vi "CalcControl.vi"(4 "Multiplier":dbl=1.0, 5 "Change Brake":dbl=0.02, 6 "Change Throttle":dbl=0.02, 7 "Current Speed":dbl format="%#_13g", 8 "Set Speed":dbl=1.0 format="%#_13g", 9 "Deadzone":dbl=0.01 format="%#_13g", 10 "Current Brake":dbl=0.5499999999999999 format="%#_13g", 11 "Current Throttle":dbl=0.45 format="%#_13g") -> (1 "Change?":bool=TRUE, 2 "New Brake":dbl=0.49999999999999994 format="%#_13g", 3 "New Throttle":dbl=0.5 format="%#_13g")   [LabVIEW 2014]
panel:
  out "NaN/Path/Refnum?":bool
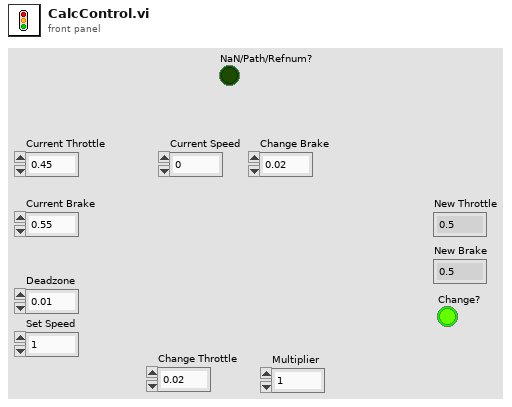
[diagram p1: front panel]
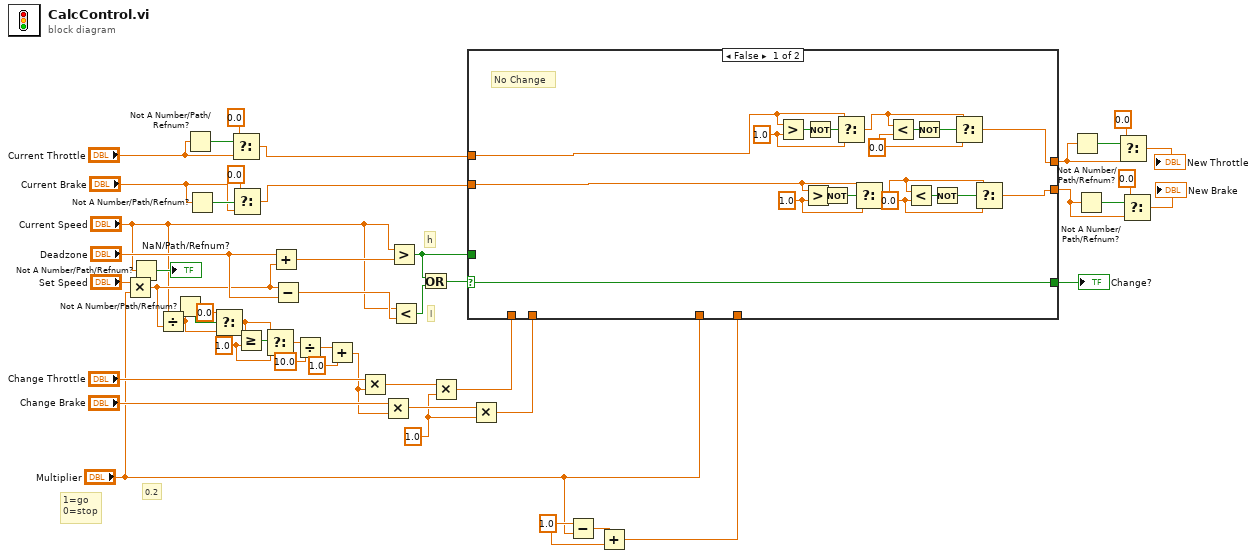
[diagram p0: block diagram]
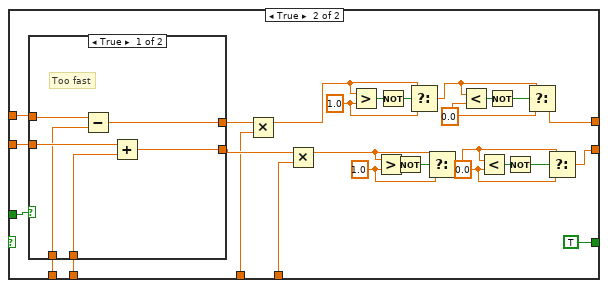
[diagram p2: hidden frame]
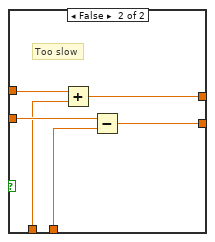
[diagram p3: hidden frame]
diagram:
  w26 = 1.0 ("y")
  w28 = 1.0 ("x")
  w40 = 1.0 ("y")
  # "0.2"
  # "1=go\n0=stop"
  # "l"
  # "h"
  n1 = Multiply(x="Set Speed", y="Multiplier") -> (x*y=w25:dbl)
  n2 = Not A Number/Path/Refnum?(number/path/refnum="Current Speed") -> (NaN/Path/Refnum?=→"NaN/Path/Refnum?":bool)
  n3 = Divide(x="Current Speed", y=w25) -> (x/y=w21:dbl)
  n4 = Not A Number/Path/Refnum?(number/path/refnum=w21) -> (NaN/Path/Refnum?=w23:bool)
  n5 = Not A Number/Path/Refnum?(number/path/refnum="Current Throttle") -> (NaN/Path/Refnum?=w19:bool)
  n6 = Not A Number/Path/Refnum?(number/path/refnum="Current Brake") -> (NaN/Path/Refnum?=w18:bool)
  n7 = Select(t=0.0, s=w23, f=w21) -> (s? t:f=w22:dbl)
  n8 = Select(t=0.0, s=w19, f="Current Throttle") -> (s? t:f=w14:dbl)
  n9 = Select(t=0.0, s=w18, f="Current Brake") -> (s? t:f=w16:dbl)
  n10 = Greater Or Equal?(x=w22, y=w40) -> (x >= y?=w39:bool)
  n11 = Select(t=w22, s=w39, f=w40) -> (s? t:f=w37:dbl)
  n12 = Add(x="Deadzone", y=w25) -> (x+y=w48:dbl)
  n13 = Subtract(x=w25, y="Deadzone") -> (x-y=w47:dbl)
  n14 = Divide(x=w37, y=10.0) -> (x/y=w38:dbl)
  n15 = Add(x=w38, y=1.0) -> (x+y=w34:dbl)
  n16 = Multiply(x="Change Throttle", y=w34) -> (x*y=w31:dbl)
  n17 = Multiply(x="Change Brake", y=w34) -> (x*y=w33:dbl)
  n18 = Greater?(x="Current Speed", y=w48) -> (0:w44:bool)
  n19 = Less?(x="Current Speed", y=w47) -> (x < y?=w46:bool)
  n20 = Or(x=w44, y=w46) -> (x .or. y?=w45:bool)
  n21 = Multiply(x=w31, y=w26) -> (x*y=w30:dbl)
  n22 = Multiply(x=w33, y=w26) -> (x*y=w32:dbl)
  n23 = Subtract(x=w28, y="Multiplier") -> (x-y=w29:dbl)
  n24 = Add(x=w29, y=w28) -> (x+y=w27:dbl)
  n25 = case shown="False" w45 {
    selector: w45 -> [w68 _]
    tunnel: w44 -> [_ w96]
    tunnel: w14 -> [w52 w95]
    tunnel: w16 -> [w53 w94]
    tunnel: w30 -> [_ w93]
    tunnel: [w51 w75] -> w3
    tunnel: [w50 w74] -> w4
    tunnel: [w68 TRUE] -> w43
    tunnel: w32 -> [_ w73]
    tunnel: w27 -> [_ w70]
    tunnel: "Multiplier" -> [_ w69]
    frame False {
      w62 = 0.0 ("y")
      w61 = 1.0 ("y")
      w65 = 0.0 ("y")
      w66 = 1.0 ("y")
      # "No Change"
      n26 = Greater?(x=w52, y=w66) -> (0:w67:bool)
      n27 = Greater?(x=w53, y=w61) -> (0:w60:bool)
      n28 = Not(x=w67) -> (.not. x?=w54:bool)
      n29 = Not(x=w60) -> (.not. x?=w56:bool)
      n30 = Select(t=w52, s=w54, f=w66) -> (s? t:f=w58:dbl)
      n31 = Select(t=w53, s=w56, f=w61) -> (s? t:f=w59:dbl)
      n32 = Less?(x=w58, y=w65) -> (x < y?=w64:bool)
      n33 = Less?(x=w59, y=w62) -> (x < y?=w63:bool)
      n34 = Not(x=w64) -> (.not. x?=w55:bool)
      n35 = Not(x=w63) -> (.not. x?=w57:bool)
      n36 = Select(t=w58, s=w55, f=w65) -> (s? t:f=w51:dbl)
      n37 = Select(t=w59, s=w57, f=w62) -> (s? t:f=w50:dbl)
    }
    frame True {
      w86 = 0.0 ("y")
      w85 = 1.0 ("y")
      w89 = 0.0 ("y")
      w90 = 1.0 ("y")
      n38 = case shown="True" w96 {
        tunnel: w95 -> [w102 w108]
        tunnel: w94 -> [w100 w106]
        tunnel: w93 -> [w99 w105]
        tunnel: [w101 w107] -> w76
        tunnel: [w98 w104] -> w77
        tunnel: w73 -> [w97 w103]
        frame True {
          # "Too fast"
          n39 = Subtract(x=w102, y=w99) -> (x-y=w101:dbl)
          n40 = Add(x=w100, y=w97) -> (x+y=w98:dbl)
        }
        frame False {
          # "Too slow"
          n41 = Add(x=w108, y=w105) -> (x+y=w107:dbl)
          n42 = Subtract(x=w106, y=w103) -> (x-y=w104:dbl)
        }
      }
      n43 = Multiply(x=w76, y=w69) -> (x*y=w72:dbl)
      n44 = Multiply(x=w77, y=w70) -> (x*y=w71:dbl)
      n45 = Greater?(x=w72, y=w90) -> (0:w91:bool)
      n46 = Greater?(x=w71, y=w85) -> (0:w84:bool)
      n47 = Not(x=w91) -> (.not. x?=w78:bool)
      n48 = Not(x=w84) -> (.not. x?=w80:bool)
      n49 = Select(t=w72, s=w78, f=w90) -> (s? t:f=w82:dbl)
      n50 = Select(t=w71, s=w80, f=w85) -> (s? t:f=w83:dbl)
      n51 = Less?(x=w82, y=w89) -> (x < y?=w88:bool)
      n52 = Less?(x=w83, y=w86) -> (x < y?=w87:bool)
      n53 = Not(x=w88) -> (.not. x?=w79:bool)
      n54 = Not(x=w87) -> (.not. x?=w81:bool)
      n55 = Select(t=w82, s=w79, f=w89) -> (s? t:f=w75:dbl)
      n56 = Select(t=w83, s=w81, f=w86) -> (s? t:f=w74:dbl)
    }
  }
  "Change?" <- w43
  n57 = Not A Number/Path/Refnum?(number/path/refnum=w3) -> (NaN/Path/Refnum?=w7:bool)
  n58 = Not A Number/Path/Refnum?(number/path/refnum=w4) -> (NaN/Path/Refnum?=w6:bool)
  n59 = Select(t=0.0, s=w7, f=w3) -> (s? t:f=→"New Throttle":dbl)
  n60 = Select(t=0.0, s=w6, f=w4) -> (s? t:f=→"New Brake":dbl)
